vi "get channels test.vi"() -> ()   [LabVIEW 2014, in "FPGA Windows Tests.lvlib"]
doc: "Tests the 'Get Channels' VI of the Configuration class."
uses:
  FPGA Windows Tests.lvlib
  module/configuration/FPGA Module configuration.lvclass
panel:
  out "error out":errorcluster
  out "channels match":bool
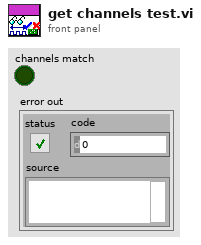
[diagram p1: front panel]
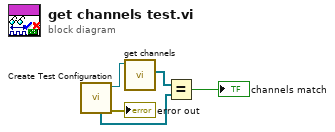
[diagram p0: block diagram]
diagram:
  n1 = call "Create Test Configuration.vi"() -> ("error out"=→"error out":errorcluster, "Module Configuration"=w3:refnum<class "FPGA Module configuration.lvclass">, "Channels"=w1:refnum<class "TBM channel.lvclass">[])  [unwired: 6 in, 3 out]
  n2 = call-dynamic "get channels.vi"("FPGA Module configuration in"=w3) -> ("channels"=w5:refnum<class "TBM channel.lvclass">[])  [unwired: 9 in, 1 out]
  n3 = Equal?(x=w5, y=w1) -> (x = y?=→"channels match":bool)
